vi "Read text from the Windows clipboard.vi"(8 "Error In":errorcluster) -> (0 "Error out":errorcluster, 2 "Clipboard data available?":bool, 3 "Text from clipboard":string="\r\n")   [LabVIEW 2013]
doc: "Use Windows DLL calls to read text from the clipboard.\n\nDr. Chris Empson\nSchool of Chemistry\nUniversity of Leeds\nUK\n\nc.j.empson@leeds.ac.uk\nTwitter: @monty_mcmont\nDownloaded from https://github.com/mcmont/LabVIEW_examples"
panel:
  # "Read text from the Windows clipboard.\n\nDr. Chris Empson\nSchool of Chemistry\nUniversity of Leeds\nUK\n\nc.j.empson@leeds.ac.uk\nTwitter: @monty_mcmont\nDownloaded from https://github.com/mcmont/LabVIEW_examples"
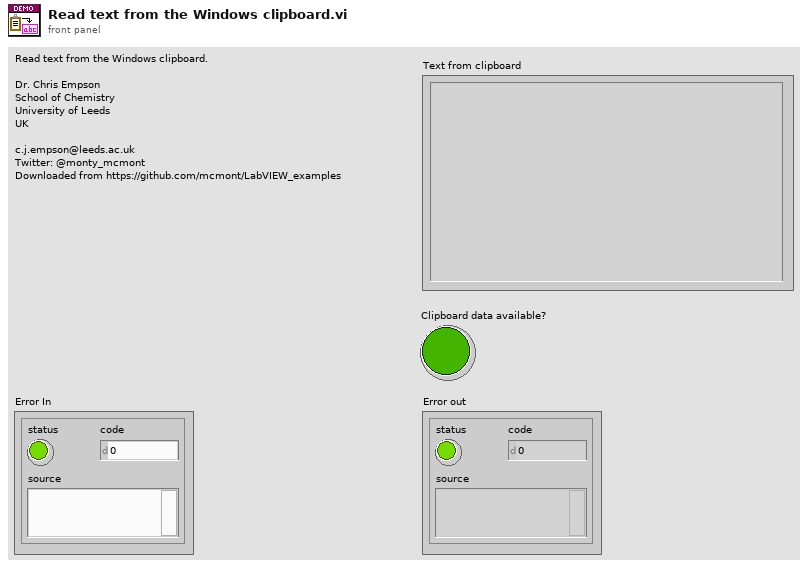
[diagram p1: front panel]
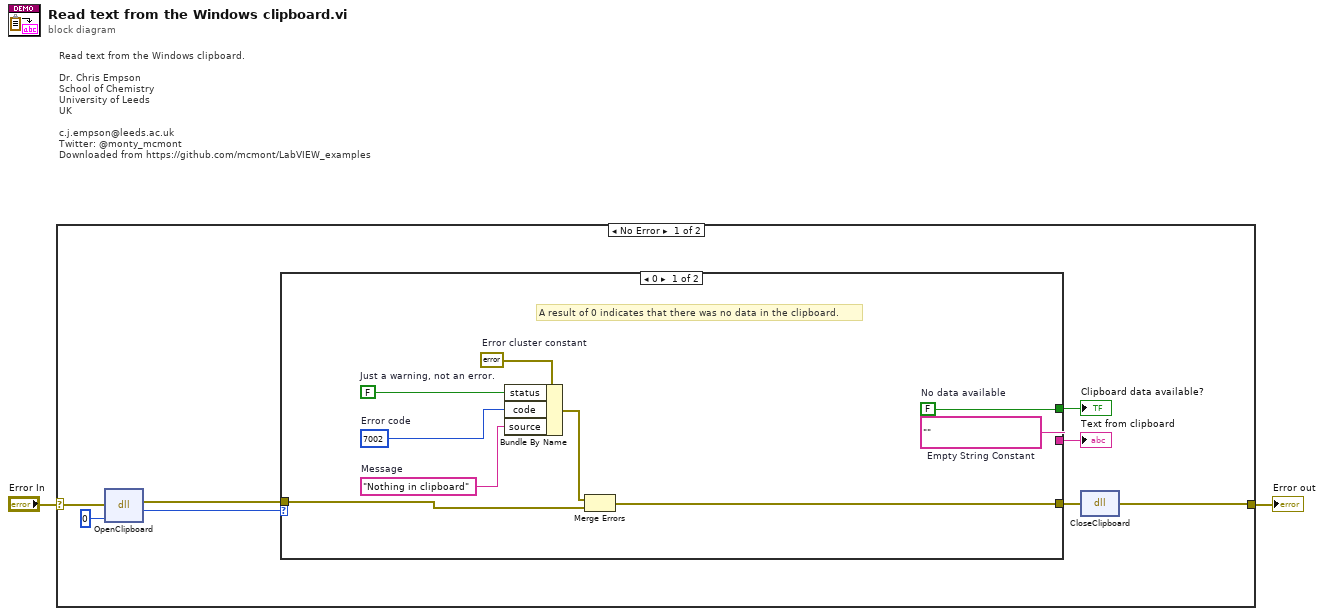
[diagram p0: block diagram]
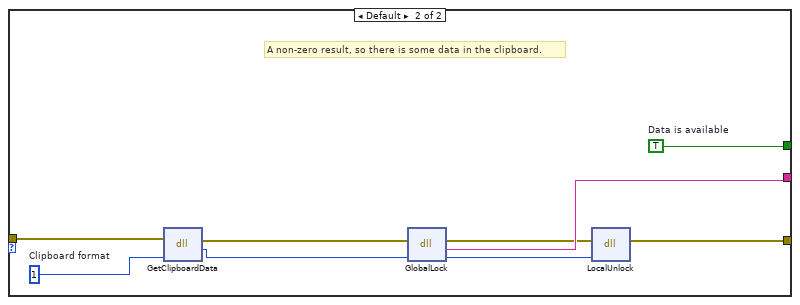
[diagram p2: hidden frame]
diagram:
  # "Read text from the Windows clipboard.\n\nDr. Chris Empson\nSchool of Chemistry\nUniversity of Leeds\nUK\n\nc.j.empson@leeds.ac.uk\nTwitter: @monty_mcmont\nDownloaded from https://github.com/mcmont/LabVIEW_examples"
  n1 = case shown="No Error" "Error In" {
    selector: "Error In" -> [w7 w29]
    tunnel: [w3 w29] -> w2
    frame No Error {
      n2 = dll-call lib="user32" fn="OpenClipboard" label="Call user32.dll : OpenClipboard"(error in=w7, "owner"=0) -> (error out=w5:errorcluster, w9:i32)  [unwired: 3 in, 1 out]
      n3 = case shown="0" w9 {
        tunnel: [w19 w25] -> w8
        tunnel: [w16 w20] -> w6
        tunnel: w5 -> [w12 w22]
        tunnel: [w11 w21] -> w4
        frame 0 {
          w14 = FALSE  # Just a warning, not an error.
          w15 = errorcluster {"status"=FALSE, "code"=0, "source"=""}  # Error cluster constant
          w16 = FALSE  # No data available
          w17 = 7002  # Error code
          w18 = "Nothing in clipboard"  # Message
          w19 = ""  # Empty String Constant
          # "A result of 0 indicates that there was no data in the clipboard."
          n4 = Bundle By Name(cluster=w15, "status"=w14, "code"=w17, "source"=w18) -> (w13:errorcluster)
          n5 = Merge Errors(w13, w12) -> (w11:errorcluster)
        }
        frame Default {
          w20 = TRUE  # Data is available
          w28 = 1  # Clipboard format
          # "Text format. Each line ends with a carriage return/linefeed (CR-LF) combination. Full list of clipboard formats:\nhttps://msdn.microsoft.com/en-us/library/windows/desktop/ms649013(v=vs.85).aspx#_win32_Standard_Clipboard_Formats"
          # "A non-zero result, so there is some data in the clipboard."
          n6 = dll-call lib="user32" fn="GetClipboardData" label="Call user32.dll : GetClipboardData"(error in=w22, "uFormat"=w28) -> (error out=w24:errorcluster, w27:i32)  [unwired: 3 in, 1 out]
          n7 = dll-call lib="kernel32" fn="GlobalLock" label="Call kernel32.dll : GlobalLock"(error in=w24, "hGlobalMemory"=w27) -> (error out=w23:errorcluster, w25:string, "hGlobalMemory"=w26:i32)  [unwired: 2 in, 1 out]
          n8 = dll-call lib="kernel32" fn="LocalUnlock" label="Call kernel32.dll : LocalUnlock"(error in=w23, "hGlobalMemory"=w26) -> (error out=w21:errorcluster)  [unwired: 4 in, 1 out]
        }
      }
      "Text from clipboard" <- w8
      "Clipboard data available?" <- w6
      n9 = dll-call lib="user32" fn="CloseClipboard" label="Call user32.dll : CloseClipboard"(error in=w4) -> (error out=w3:errorcluster)  [unwired: 3 in, 1 out]
    }
    frame Error {
    }
  }
  "Error out" <- w2
